vi "show file in explorer.vi"(8 "error in (no error)":errorcluster, 11 "Julia user functions script":path=path "C:/_LabView_projects/ZMQ/LV_ZMQ_Jl.jl/src/Julia/dummy.jl") -> (0 "error out":errorcluster, 3 "return code":i32)   [LabVIEW 2018, in "LV-0mq-Julia_roundtrip-lib.lvlib"]
uses:
  LV-0mq-Julia_roundtrip-lib.lvlib
panel:
  out "tmp file":path
  out "Julia script":string
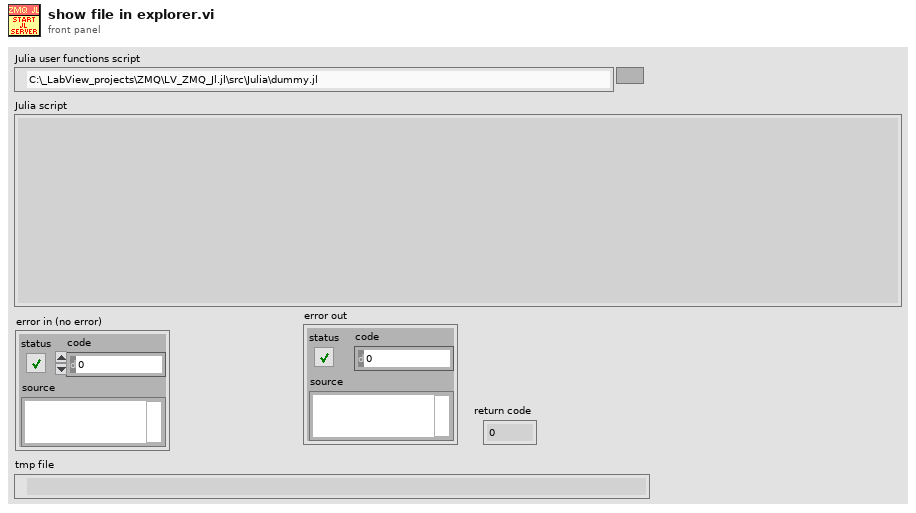
[diagram p1: front panel]
types:
  T1 = enum16{"open", "replace", "create", "open or create", "replace or create", "replace or create with confirmation"}
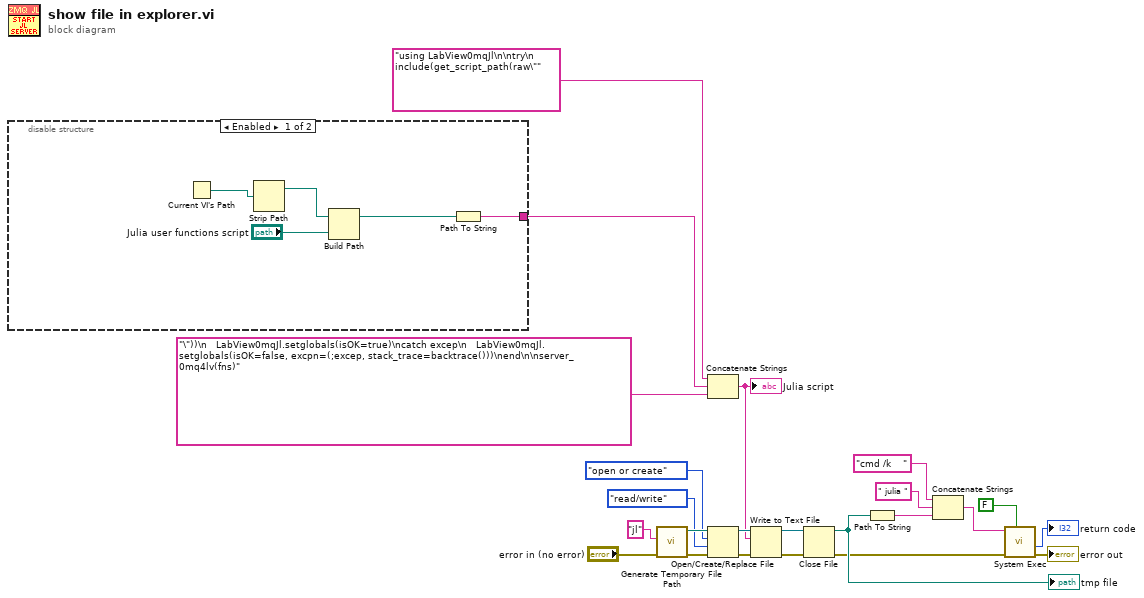
[diagram p0: block diagram]
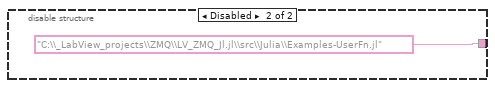
[diagram p2: hidden frame]
diagram:
  n1 = disable-structure shown="Enabled" {
    disable-tunnel: [w28 "C:\\_LabView_projects\\ZMQ\\LV_ZMQ_Jl.jl\\src\\Julia\\Examples-UserFn.jl"] -> w21
    frame Enabled {
      n2 = Current VI's Path() -> (path=w27:path)
      n3 = Strip Path(path=w27) -> (stripped path=w26:path)  [unwired: 1 out]
      n4 = Build Path(base path=w26, name or relative path="Julia user functions script") -> (appended path=w25:path)
      n5 = Path To String(path=w25) -> (string=w28:string)
    }
    frame Disabled {
    }
  }
  n6 = call <vilib>:"Generate Temporary File Path.vi"("error in (no error)"="error in (no error)", "Temporary File Extension (tmp)"="jl") -> ("error out"=w18:errorcluster, "Unique Temporary File Path"=w19:path)  [unwired: 8 in]
  n7 = Concatenate Strings("using LabView0mqJl\n\ntry\n   include(get_script_path(raw\"", w21, "\"))\n   LabView0mqJl.setglobals(isOK=true)\ncatch excep\n   LabView0mqJl.setglobals(isOK=false, excpn=(;excep, stack_trace=backtrace()))\nend\n\nserver_0mq4lv(fns)") -> (w13:string)
  "Julia script" <- w13
  n8 = Open/Create/Replace File(file path (use dialog)=w19, error in=w18, operation (0:open)=T1."open or create", access (0:read/write)=enum16{"read/write", "read-only", "write-only"}."read/write") -> (refnum out=w14:refnum<file>, error out=w15:errorcluster)  [unwired: 2 in, 1 out]
  n9 = Write to Text File(file (use dialog)=w14, text=w13, error in=w15) -> (refnum out=w12:refnum<file>, error out=w11:errorcluster)  [unwired: 1 in, 1 out]
  n10 = Close File(refnum=w12, error in=w11) -> (path=w3:path, error out=w1:errorcluster)
  "tmp file" <- w3
  n11 = Path To String(path=w3) -> (string=w7:string)
  n12 = Concatenate Strings("cmd /k    ", " julia ", w7) -> (w6:string)
  n13 = call <vilib>:"System Exec.vi"("wait until completion? (T)"=FALSE, "error in (no error)"=w1, "command line"=w6) -> ("error out"=→"error out":errorcluster, "return code"=→"return code":i32)  [unwired: 5 in, 2 out]
